vi "Insert Theme List in Menu.vi"(8 "error in (no error)":errorcluster, 11 "Menu in":refnum<k9>) -> (0 "error out":errorcluster)   [LabVIEW 2021, in "Notebook.lvlib"]
uses:
  Notebook.lvlib
  Notebook Parameters List.ctl
  Notebook Theme.ctl
  Rich Text Box/Named Text Style.ctl
  Rich Text Box/Text Formatting.ctl
  Rich Text Box/Text Colors.ctl
  Rich Text Box/Text Style.ctl
  Rich Text Box/Text Alignment.ctl
  Rich Text Box/Rich Text Box.lvlib
panel:
  # "see the License on the block diagram (Ctrl+E or Window:Show Block Diagram)"
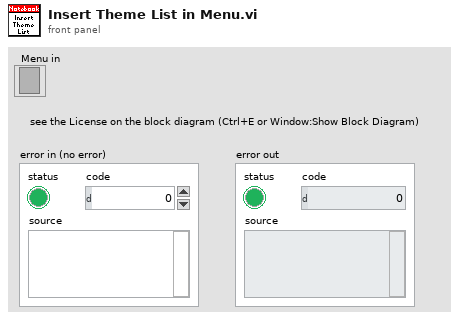
[diagram p1: front panel]
types:
  T1 = typedef "Notebook.lvlib/Notebook Theme.ctl" = cluster{"Theme Name":string, "[Named Text Styles]":T2[], "Page Color":T4}
  T2 = typedef "Notebook.lvlib/Named Text Style.ctl" = cluster{"Text Formatting":T3, "Text Style Name":string}
  T3 = typedef "Rich Text Box.lvlib/Text Formatting.ctl" = cluster{"Font":string, "Text Color":T4, "Background Color":T4, "Style":T5, "Font Size":dbl, "Alignment":T6}
  T4 = typedef "Rich Text Box.lvlib/Text Colors.ctl" = enum16{"Unchanged", "Black", "Blue", "Cyan", "Maroon", "Gray", "Violet", "Green", "Light Green", "Orange", "Yellow", "Magenta", "Red", "White"}
  T5 = typedef "Rich Text Box.lvlib/Text Style.ctl" = enum16{"Regular", "Bold", "Italic", "Underline", "Strikeout"}
  T6 = typedef "Rich Text Box.lvlib/Text Alignment.ctl" = enum16{"Left", "Right", "Center"}
  T7 = typedef "Notebook.lvlib/Notebook Parameters List.ctl" = enum16{"First Opening?", "Saved Notebook?", "Saved Notebook Path", "Beep on Error?", "Notebook Themes", "Current Theme Name"}
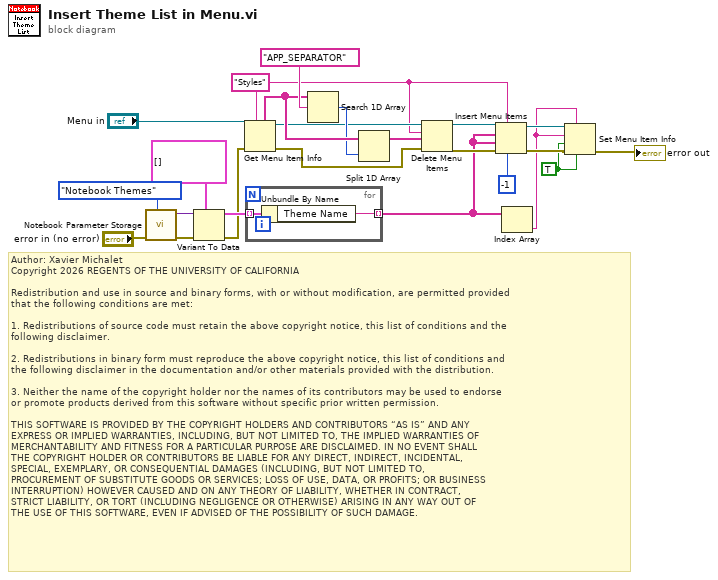
[diagram p0: block diagram]
diagram:
  w3 = TRUE ("enabled")
  w12 = "Styles" ("item tag")
  # "Author: Xavier Michalet\nCopyright 2026 REGENTS OF THE UNIVERSITY OF CALIFORNIA\n\nRedistribution and use in source and binary forms, with or without modification, are permitted provided\nthat the following conditions are met:\n\n1. Redistributions of source code must retain the above copyright notice, this list of conditions and the\nfollowing disclaimer.\n\n2. Redistributions in binary form must reproduce the above copyright notice, this list of conditions and\nthe following disclaimer in the documentation and/or other materials provided with the distribution.\n\n3. Neither the name of the copyright holder nor the names of its contributors may be used to endorse \nor promote products derived from this software without specific prior written permission.\n\nTHIS SOFTWARE IS PROVIDED BY THE COPYRIGHT HOLDERS AND CONTRIBUTORS “AS IS” AND ANY \nEXPRESS OR IMPLIED WARRANTIES, INCLUDING, BUT NOT LIMITED TO, THE IMPLIED WARRANTIES OF\nMERCHANTABILITY AND FITNESS FOR A PARTICULAR PURPOSE ARE DISCLAIMED. IN NO EVENT SHALL\nTHE COPYRIGHT HOLDER OR CONTRIBUTORS BE LIABLE FOR ANY DIRECT, INDIRECT, INCIDENTAL, \nSPECIAL, EXEMPLARY, OR CONSEQUENTIAL DAMAGES (INCLUDING, BUT NOT LIMITED TO, \nPROCUREMENT OF SUBSTITUTE GOODS OR SERVICES; LOSS OF USE, DATA, OR PROFITS; OR BUSINESS\nINTERRUPTION) HOWEVER CAUSED AND ON ANY THEORY OF LIABILITY, WHETHER IN CONTRACT, \nSTRICT LIABILITY, OR TORT (INCLUDING NEGLIGENCE OR OTHERWISE) ARISING IN ANY WAY OUT OF\nTHE USE OF THIS SOFTWARE, EVEN IF ADVISED OF THE POSSIBILITY OF SUCH DAMAGE."
  n1 = call "Notebook Parameter Storage.vi"("Notebook Parameter List"=Notebook_Parameters_List."Notebook Themes", "Error In"="error in (no error)") -> ("Error Out"=w22:errorcluster, "Data out"=w23:variant)  [unwired: 8 in]
  n2 = Variant To Data(error in=w22, type=T1[] [] ("Array"), Variant=w23) -> (data=w9:T1[], error out=w7:errorcluster)
  n3 = Get Menu Item Info(7:w12, 8:w7, 11:"Menu in") -> (0:w14:errorcluster, 3:w15:refnum<k9>, 5:w18:string[])  [unwired: 4 out]
  n4 = for {
    tunnel: w9 -> [w26] mode=indexing
    tunnel: [w25] -> w4 mode=indexing
    n5 = Unbundle By Name(w26) -> ("Theme Name"=w25:string)
  }
  n6 = Search 1D Array(1D array=w18, element="APP_SEPARATOR") -> (index of element=w17:i32)  [unwired: 1 in]
  n7 = Split 1D Array(array=w18, index=w17) -> (first subarray=w16:string[])  [unwired: 1 out]
  n8 = Delete Menu Items(6:w14, 7:w16, 8:w12, 9:w15) -> (0:w11:errorcluster, 3:w13:refnum<k9>)
  n9 = Insert Menu Items(4:-1, 5:w12, 6:w11, 7:w4, 8:w4, 9:w13) -> (0:w5:errorcluster, 3:w6:refnum<k9>)  [unwired: 1 out]
  n10 = Index Array(array=w4) -> (element=w1:string)  [unwired: 1 in]
  n11 = Set Menu Item Info(6:w3, 7:w1, 8:w5, 9:w3, 10:w1, 11:w6) -> (0:→"error out":errorcluster)  [unwired: 1 in, 1 out]
